vi "DAQ_continuous_output_test.vi"() -> ()   [LabVIEW 2017]
uses:
  <vilib>/Utility/error.llb/DialogType.ctl
  <vilib>/DAQmx/write.llb/DAQmx Write (Analog Wfm 1Chan NSamp).vi
  <vilib>/DAQmx/create/channels.llb/DAQmx Create Channel (AO-Voltage-Basic).vi
  <vilib>/DAQmx/configure/timing.llb/DAQmx Timing (Sample Clock).vi
  <vilib>/DAQmx/miscellaneous.llb/DAQmx Fill In Error Info.vi
  <resource>/objmgr/daqmx.rc
  <vilib>/measure/NI_MABase.lvlib
panel:
  in  "Frequency, Hz":dbl=10000.0 format="%0.1p"
  in  "Amplitude, V":dbl=0.5 format="%0.3f"
  out "Waveform Graph":waveform(dbl)(graph)={"t0"=timestamp(0 s since 1904-01-01), "dt"=2e-06, "Y"=array[10000 elements]}
  in  "Physical Channel":tag="DAQ6363/ao0"
  out "Actual Sample Rate":dbl=500000.0 format="%0.2f"
  in  "Stop":bool
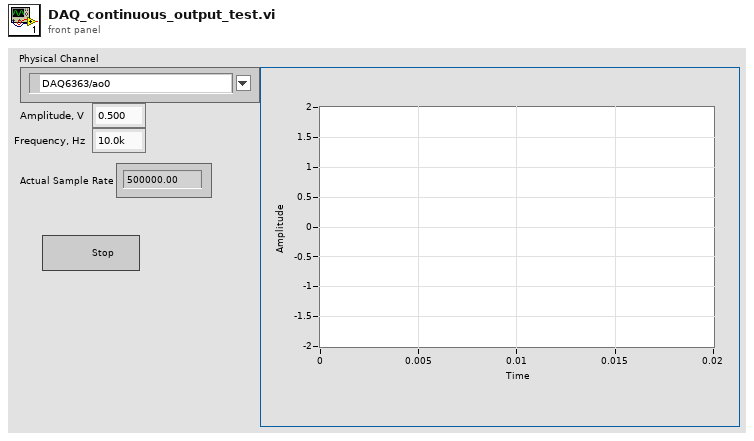
[diagram p1: front panel]
types:
  T1 = enum16{"Sine Wave", "Triangle Wave", "Square Wave", "Sawtooth Wave"}
  T2 = typedef "DialogType.ctl" = u16
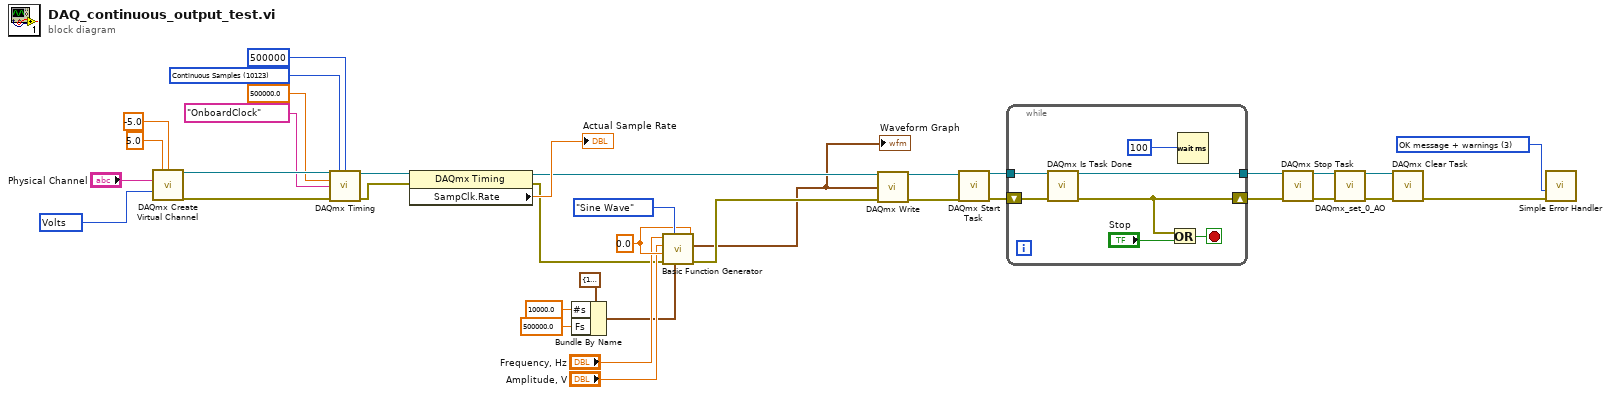
[diagram p0: block diagram]
diagram:
  w8 = 10348 items=["Volts"=10348, "From Custom Scale"=10065] ("units")
  w19 = 0.0 ("phase")
  w25 = T2 3 items=["no dialog", "OK message", "continue or stop message", "OK message + warnings", "continue/stop + warnings"] ("type of dialog (OK msg:1)")
  w35 = 10123 items=["Finite Samples"=10178, "Continuous Samples"=10123, "Hardware Timed Single Point"=12522] ("Sample Mode")
  n1 = call-poly <vilib>:"DAQmx Create Virtual Channel.vi"("maximum value"=5.0, "minimum value"=-5.0, "physical channels"="Physical Channel", "units"=w8) -> ("task out"=w33:refnum<k21>, "error out"=w34:errorcluster)  [unwired: 10 in]
  n2 = call-poly <vilib>:"DAQmx Timing.vi"("task/channels in"=w33, "sample mode"=w35, "samples per channel"=500000, "rate"=500000.0, "source"=tag "OnboardClock", "error in"=w34) -> ("task out"=w37:refnum<k21>, "error out"=w36:errorcluster)  [unwired: 8 in]
  n3 = property class="DAQmx Timing"(reference=w37, error in=w36) -> (reference out=w24:refnum<k21>, error out=w16:errorcluster, "SampClk.Rate"=→"Actual Sample Rate":dbl)
  n4 = Bundle By Name(cluster=cluster{"Fs":dbl, "#s":dbl} {"Fs"=1000.0, "#s"=1000.0} ("sampling info"), "#s"=10000.0, "Fs"=500000.0) -> (w5:cluster{"Fs":dbl, "#s":dbl})
  n5 = call <vilib>:"Basic Function Generator.vi"("offset"=w19, "sampling info"=w5, "signal type"=T1."Sine Wave", "error in (no error)"=w16, "phase"=w19, "amplitude"="Amplitude, V", "frequency"="Frequency, Hz") -> ("error out"=w15:errorcluster, "signal out"=w14:waveform(dbl))  [unwired: 2 in, 1 out]
  "Waveform Graph" <- w14
  n6 = call-poly <vilib>:"DAQmx Write.vi"("task/channels in"=w24, "data"=w14, "error in"=w15) -> ("task out"=w27:refnum<k21>, "error out"=w26:errorcluster)  [unwired: 10 in, 1 out]
  n7 = call <vilib>:"DAQmx Start Task.vi"("task/channels in"=w27, "error in"=w26) -> ("task out"=w32:refnum<k21>, "error out"=w31:errorcluster)  [unwired: 12 in]
  n8 = while {
    tunnel: w32 -> [w44]
    tunnel: [w41] -> w7
    shift-right: [w39] -> w6
    shift-left: w31 -> [w43]
    stop <- w42 stop-if-true
    n9 = call <vilib>:"DAQmx Is Task Done.vi"("task/channels in"=w44, "error in"=w43) -> ("task out"=w41:refnum<k21>, "error out"=w39:errorcluster)  [unwired: 11 in, 1 out]
    n10 = Or(x=w39, y="Stop") -> (x .or. y?=w42:bool)
    n11 = Wait (ms)(milliseconds to wait=u32 100 ("millisecond multiple")) -> ()  [unwired: 1 out]
  }
  n12 = call <vilib>:"DAQmx Stop Task.vi"("task/channels in"=w7, "error in"=w6) -> ("task out"=w4:refnum<k21>, "error out"=w3:errorcluster)  [unwired: 12 in]
  n13 = call "DAQmx_set_0_AO.vi"("Refnum in"=w4, "error in (no error)"=w3) -> ("Refnum out"=w2:refnum<k21>, "error out"=w1:errorcluster)  [unwired: 12 in]
  n14 = call <vilib>:"DAQmx Clear Task.vi"("task in"=w2, "error in"=w1) -> ("error out"=w30:errorcluster)  [unwired: 13 in]
  n15 = call <vilib>:"Simple Error Handler.vi"("type of dialog (OK msg:1)"=w25, "error in (no error)"=w30) -> ()  [unwired: 3 in, 5 out]
